vi "生成校准信息.vi"(5 "量程选择":enum16{"低量程", "高量程"}(ring), 7 "公式系数":cluster{"K":string, "B":string, "X^2":string}, 8 "启用":bool[](array[boolean]), 9 "校准时间":string[](array[string]), 10 "信号值":string[](array[string]), 11 "校准浓度":string[](array[string])) -> ()   [LabVIEW 2016, in "斯坦道CODMn.lvlib"]
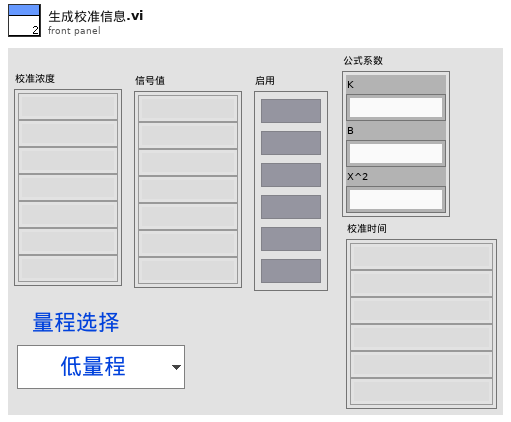
[diagram p1: front panel]
types:
  T1 = cluster{"时间标识":timestamp, "参数":string, "日志信息":string, "流程参数":string}
  T2 = cluster{"时间标识":timestamp, "设备":string, "日志信息":string, "流程参数":string}
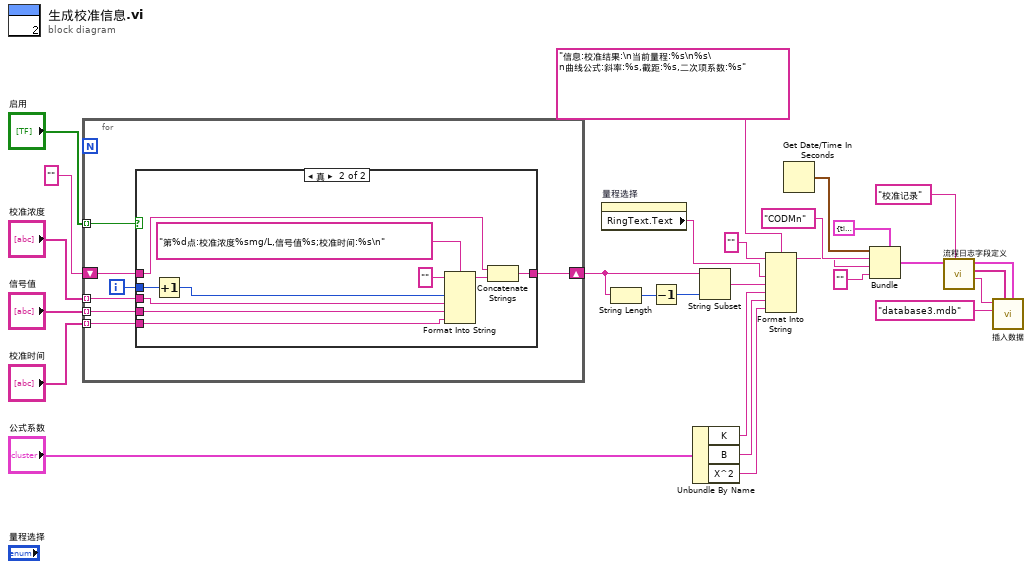
[diagram p0: block diagram]
diagram:
  n1 = for {
    tunnel: "启用" -> [w34] mode=indexing
    tunnel: "校准浓度" -> [w32] mode=indexing
    tunnel: "信号值" -> [w31] mode=indexing
    shift-right: [w30] -> w21
    shift-left: "" -> [w29]
    tunnel: "校准时间" -> [w28] mode=indexing
    i -> [w33]
    n2 = case shown="真" w34 {
      tunnel: w33 -> [_ w43]
      tunnel: w32 -> [_ w42]
      tunnel: w31 -> [_ w41]
      tunnel: [w35 w38] -> w30
      tunnel: w29 -> [w35 w37]
      tunnel: w28 -> [_ w36]
      frame False {
      }
      frame True {
        n3 = Increment(x=w43) -> (x+1=w44:i32)
        n4 = Format Into String(format string="第%d点:校准浓度%smg/L,信号值%s;校准时间:%s\n" ("格式字符串"), initial string="" ("初始字符串"), w44, w42, w41, w36) -> (resulting string=w39:string)  [unwired: 1 in, 1 out]
        n5 = Concatenate Strings(w37, w39) -> (w38:string)
      }
    }
  }
  n6 = property on="量程选择" class="Enum (严格)"() -> ("RingText.Text"=w1:string)  [unwired: 2 in, 2 out]
  n7 = String Length(string=w21) -> (length=w20:i32)
  n8 = Decrement(x=w20) -> (x-1=w19:i32)
  n9 = Unbundle By Name("公式系数") -> ("K"=w16:string, "B"=w15:string, "X^2"=w14:string)
  n10 = String Subset(string=w21, length (rest)=w19) -> (substring=w2:string)  [unwired: 1 in]
  n11 = Format Into String(format string="信息:校准结果:\n当前量程:%s\n%s\n曲线公式:斜率:%s,截距:%s,二次项系数:%s", initial string="" ("初始字符串"), w1, w2, w16, w15, w14) -> (resulting string=w3:string)  [unwired: 1 in, 1 out]
  n12 = Get Date/Time In Seconds() -> (seconds since 1Jan1904=w5:timestamp)
  n13 = Bundle(cluster=T1 {"时间标识"=timestamp(0 s since 1904-01-01), "参数"="", "日志信息"="", "流程参数"=""} ("data in"), "时间标识"=w5, "参数"="CODMn" ("table输入"), "日志信息"=w3, "流程参数"="" ("table输入")) -> (w7:T1)
  n14 = call "流程日志字段定义.vi"("table输入"="校准记录", "data in"=w7) -> ("table输出"=w11:string, "columns"=w12:string[], "data out"=w13:T2)  [unwired: 7 in]
  n15 = call "插入数据.vi"("data"=w13, "columns"=w12, "database"="database3.mdb", "table"=w11) -> ()  [unwired: 7 in, 1 out]
